vi "Score_For_Position.vi"(8 "error in (no error)":errorcluster, 10 "Elevator in":T1, 11 "Desired Floor":i32) -> (0 "error out":errorcluster, 3 "Numeric":i32)   [LabVIEW 2026]
uses:
  Controls/Door_Status_Enum.ctl
  Controls/Occupy_Status.ctl
  Controls/Floor_Status.ctl
  Controls/Motion_Status_Enum.ctl
  Controls/Car_Calls_Status.ctl
  Controls/Hall_Calls_Status.ctl
  Controls/Elevator_Status.ctl
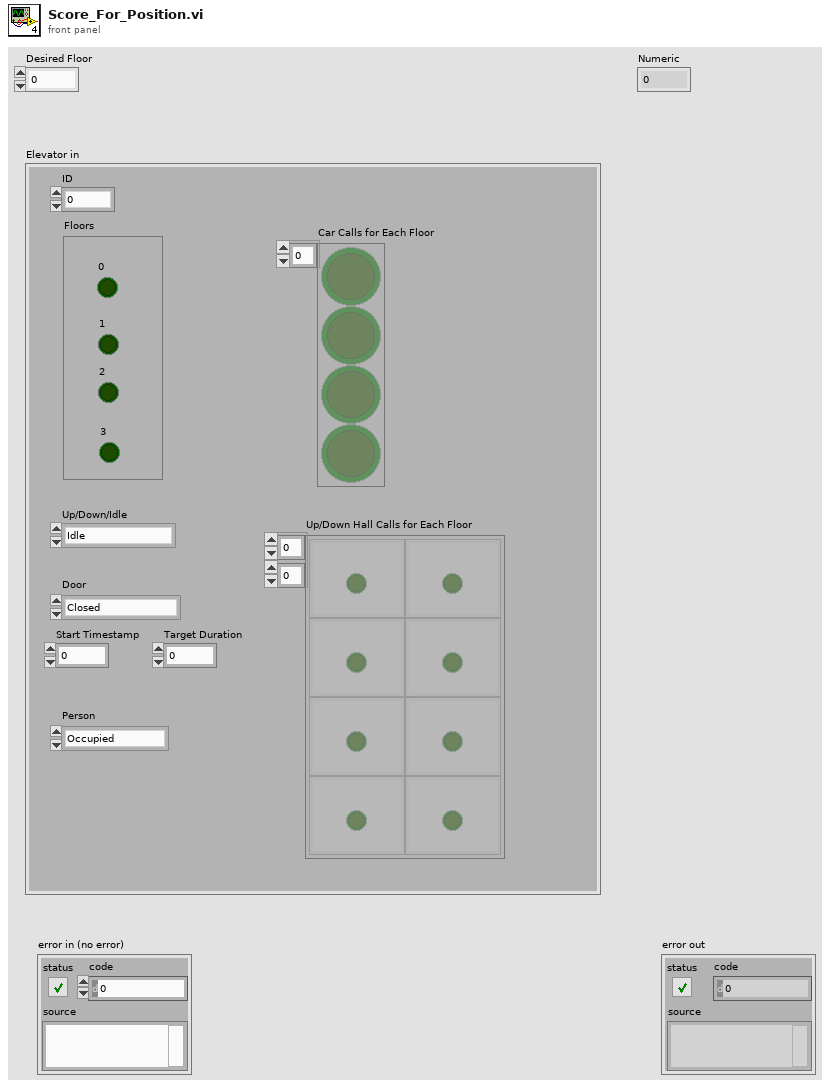
[diagram p1: front panel]
types:
  T1 = typedef "Elevator_Status.ctl" = cluster{"Door":T2, "Person":T3, "Floors":T4, "Up/Down/Idle":T5, "Car Calls for Each Floor":T6, "Up/Down Hall Calls for Each Floor":T7, "ID":i32, "Start Timestamp":u32, "Target Duration":dbl}
  T2 = typedef "Door_Status_Enum.ctl" = enum16{"Closed", "Open", "Opening", "Closing"}
  T3 = typedef "Occupy_Status.ctl" = enum16{"Occupied", "Empty"}
  T4 = typedef "Floor_Status.ctl" = cluster{"0":bool, "1":bool, "2":bool, "3":bool}
  T5 = typedef "Motion_Status_Enum.ctl" = enum16{"Idle", "Up", "Down"}
  T6 = typedef "Car_Calls_Status.ctl" = bool[]
  T7 = typedef "Hall_Calls_Status.ctl" = cluster{bool}[][]
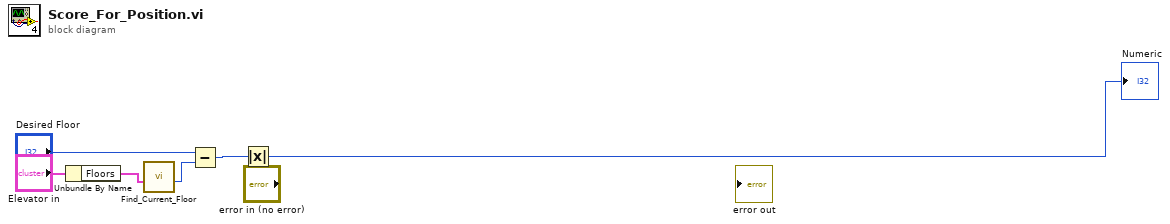
[diagram p0: block diagram]
diagram:
  n1 = Unbundle By Name("Elevator in") -> ("Floors"=w6:T4)
  n2 = call "Find_Current_Floor.vi"("Floors"=w6) -> ("Current Floor"=w4:i32)  [unwired: 7 in, 3 out]
  n3 = Subtract(x="Desired Floor", y=w4) -> (x-y=w2:i32)
  n4 = Absolute Value(x=w2) -> (abs(x)=→"Numeric":i32)
